vi "loop_shiftregister_sum_ConsNaturalNos.vi"() -> ()   [LabVIEW 2023]
panel:
  out "Numeric":dbl
  # "Random Output Set Check \n\nNumber      Sums\n5                     15\n10                    55\n20                  210"
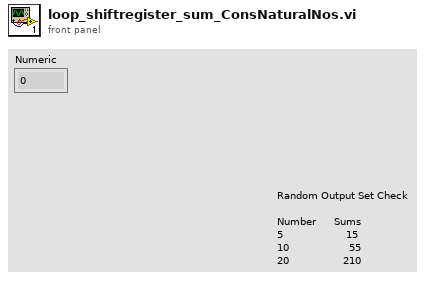
[diagram p1: front panel]
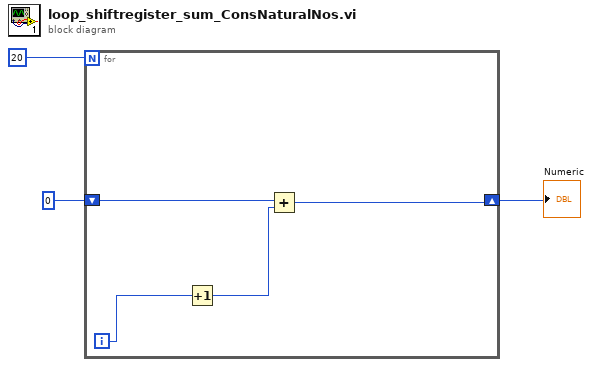
[diagram p0: block diagram]
diagram:
  n1 = for {
    N: 20 -> [_]
    shift-right: [w4] -> w1
    shift-left: 0 -> [w5]
    i -> [w7]
    n2 = Increment(x=w7) -> (x+1=w6:i32)
    n3 = Add(x=w5, y=w6) -> (x+y=w4:i32)
  }
  "Numeric" <- w1
